vi "iteracion.vi"() -> ()   [LabVIEW 2020]
panel:
  out "I":i32
  out "Number":i32
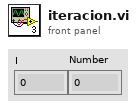
[diagram p1: front panel]
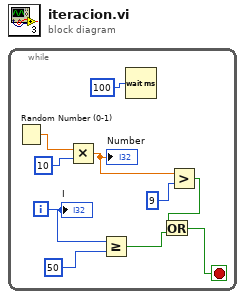
[diagram p0: block diagram]
diagram:
  n1 = while {
    i -> [w6]
    stop <- w1 stop-if-true
    n2 = Random Number (0-1)() -> (number: 0 to 1=w9:dbl)
    n3 = Multiply(x=w9, y=10) -> (x*y=w7:dbl)
    "Number" <- w7
    n4 = Greater Or Equal?(x=w6, y=50) -> (x >= y?=w2:bool)
    n5 = Wait (ms)(milliseconds to wait=100) -> ()  [unwired: 1 out]
    n6 = Greater?(x=w7, y=9) -> (0:w3:bool)
    n7 = Or(x=w3, y=w2) -> (x .or. y?=w1:bool)
    "I" <- w6
  }
